vi "0506_Definindo_ROI_esteira.vi"() -> ()   [LabVIEW 2017]
uses:
  <vilib>/userdefined/High Color/IMAQdx.ctl
  <vilib>/vision/driver/IMAQdx.llb/IMAQdx Acquisition Mode.ctl
  <vilib>/vision/driver/IMAQdx.llb/IMAQdx Buffer Number Mode.ctl
  <vilib>/vision/driver/NI_Vision_Acquisition_Software.lvlib
panel:
  out "ROI Descriptor":T1 {"Contours"."Type" items=["No Selection", "Point", "Line", "Rectangle", "Oval", "Polygon", "Freehand Region", "Annulus", "Unused2", "Unused3", "Broken Line", "Freehand Line", "Rotated Rectangle"]}
  in  "ROI Color":cluster{"Red":u8, "Green":u8, "Blue":u8}
  out "dt":dbl
  in  "Stop Button":bool
  out "Imagem Original":T2(plugin-control)
  in  "Câmera":T3="cam1"
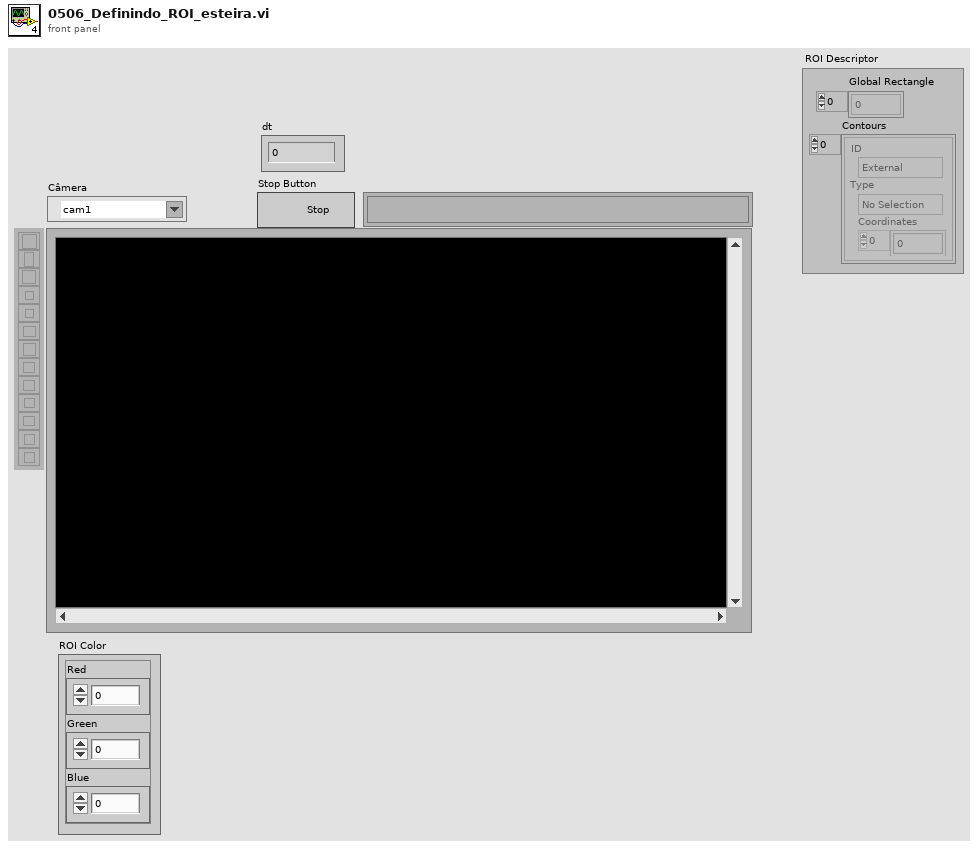
[diagram p1: front panel]
types:
  T1 = typedef "ROI Descriptor" = cluster{"Global Rectangle":i32[], "Contours":cluster{"ID":enum32{"External", "Internal"}, "Type":u32, "Coordinates":i32[]}[]}
  T2 = typedef "IMAQ Image.ctl" = refnum<image>
  T3 = typedef "IMAQdx.ctl" = refnum<k21>
  T4 = typedef "NI_Vision_Acquisition_Software.lvlib/IMAQdx Acquisition Mode.ctl" = enum32{"One Shot", "Continuous"}
  T5 = typedef "NI_Vision_Acquisition_Software.lvlib/IMAQdx Buffer Number Mode.ctl" = enum32{"Next", "Last", "Buffer Number", "Every", "Last New"}
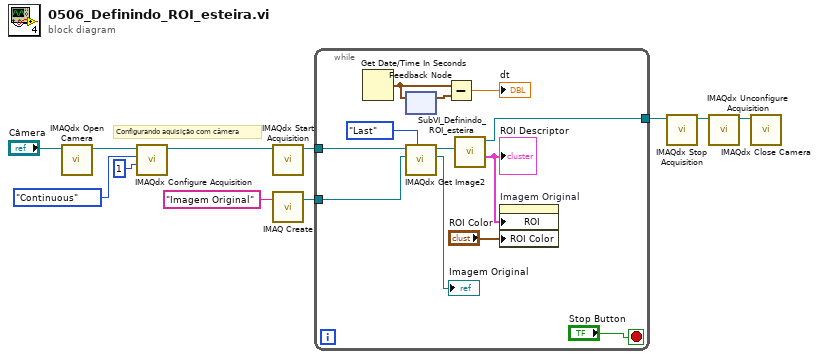
[diagram p0: block diagram]
diagram:
  # "Configurando aquisição com câmera"
  n1 = call <vilib>:"IMAQdx Open Camera.vi"("Session In"="Câmera") -> ("Session Out"=w11:T3)  [unwired: 9 in, 1 out]
  n2 = call <vilib>:"IMAQdx Configure Acquisition.vi"("Number of Buffers"=u32 1, "Continuous?"=IMAQdx_Acquisition_Mode."Continuous", "Session In"=w11) -> ("Session Out"=w10:T3)  [unwired: 7 in, 1 out]
  n3 = call <vilib>:"IMAQdx Start Acquisition.vi"("Session In"=w10) -> ("Session Out"=w4:T3)  [unwired: 9 in, 1 out]
  n4 = call "IMAQ Create"("Image Name"="Imagem Original") -> ("New Image"=w7:T2)  [unwired: 4 in, 1 out]
  n5 = while {
    tunnel: w7 -> [w23]
    tunnel: w4 -> [w21]
    tunnel: [w12] -> w1
    stop <- "Stop Button" stop-if-true
    n6 = Get Date/Time In Seconds() -> (seconds since 1Jan1904=w18:timestamp)
    n7 = feedback-in #1(w18) -> ()
    n8 = feedback #1() -> (w20:timestamp)  [unwired: 1 in]
    n9 = call <vilib>:"IMAQdx Get Image2.vi"("Buffer Number Mode (Next)"=IMAQdx_Buffer_Number_Mode."Last", "Image In"=w23, "Session In"=w21) -> ("Image Out"=→"Imagem Original":T2, "Session Out"=w13:T3)  [unwired: 5 in, 2 out]
    n10 = Subtract(x=w18, y=w20) -> (x-y=→"dt":dbl)
    n11 = call "SubVI_Definindo_ROI_esteira.vi"("Session in"=w13) -> ("ROI Descriptor"=w14:T1, "Session Out"=w12:T3)  [unwired: 8 in, 1 out]
    "ROI Descriptor" <- w14
    n12 = property on="Imagem Original" class="ImageControl"("ROI"=w14, "ROI Color"="ROI Color") -> ()  [unwired: 2 in, 2 out]
  }
  n13 = call <vilib>:"IMAQdx Stop Acquisition.vi"("Session In"=w1) -> ("Session Out"=w3:T3)  [unwired: 9 in, 1 out]
  n14 = call <vilib>:"IMAQdx Unconfigure Acquisition.vi"("Session In"=w3) -> ("Session Out"=w2:T3)  [unwired: 9 in, 1 out]
  n15 = call <vilib>:"IMAQdx Close Camera.vi"("Session In"=w2) -> ()  [unwired: 10 in, 1 out]
